vi "Lvi Board Properties.vi"(8 "error in (no error)":errorcluster, 11 "TaskRef":i32) -> (0 "error out":errorcluster, 1 "DeviceName":string, 2 "BoardModelName":string, 3 "TaskRef out":i32, 4 "DriverVersion":string, 5 "DriverName":string, 7 "function return":u32(ring))   [LabVIEW 2022 SP3, in "DtLvLink.lvlib"]
doc: "Calls directly into the entry points of the DLL of the Data Acq SDK to return information about the device. This VI is used by the higher-level VI, DtOLGetBoard."
uses:
  DtLvLink.lvlib
  <userlib>/LV-Link3/DtLvLink_64.dll
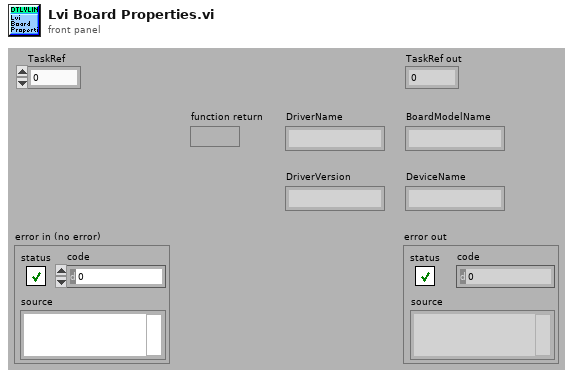
[diagram p1: front panel]
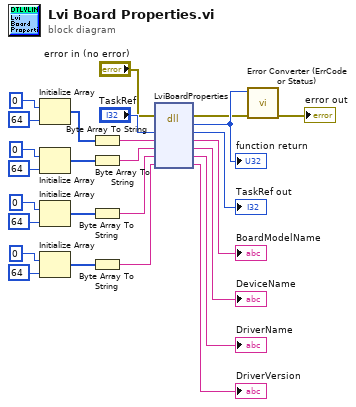
[diagram p0: block diagram]
diagram:
  n1 = Initialize Array(u8 0 ("element"), 64 ("dimension size")) -> (w23:u8[])
  n2 = Initialize Array(u8 0 ("element"), 64 ("dimension size")) -> (w18:u8[])
  n3 = Initialize Array(u8 0 ("element"), 64 ("dimension size")) -> (w13:u8[])
  n4 = Initialize Array(u8 0 ("element"), 64 ("dimension size")) -> (w8:u8[])
  n5 = Byte Array To String(unsigned byte array=w23) -> (string=w22:string)
  n6 = Byte Array To String(unsigned byte array=w18) -> (string=w17:string)
  n7 = Byte Array To String(unsigned byte array=w13) -> (string=w12:string)
  n8 = Byte Array To String(unsigned byte array=w8) -> (string=w7:string)
  n9 = dll-call lib="C:/Program Files/National Instruments/LabVIEW 2022/user.lib/LV-Link3/DtLvLink_64.*" fn="LviBoardProperties"(error in="error in (no error)", "TaskRef"="TaskRef", "BoardModelName"=w22, "DeviceName"=w17, "DriverName"=w12, "DriverVersion"=w7) -> (error out=w2:errorcluster, w26:u32, "TaskRef"=→"TaskRef out":i32, "BoardModelName"=→"BoardModelName":string, "DeviceName"=→"DeviceName":string, "DriverName"=→"DriverName":string, "DriverVersion"=→"DriverVersion":string)  [unwired: 2 in, 1 out]
  "function return" <- w26
  n10 = call "Error Converter (ErrCode or Status).vi"("error in (no error)"=w2, "error code"=w26) -> ("error out"=→"error out":errorcluster)  [unwired: 9 in]
